vi "String2Array.vi"(7 "dimension size":i32=6, 10 "String":string) -> (2 "Array":dbl[](array[numeric]))   [LabVIEW 2013]
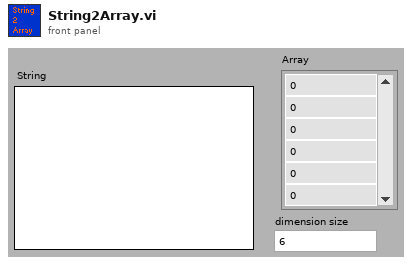
[diagram p1: front panel]
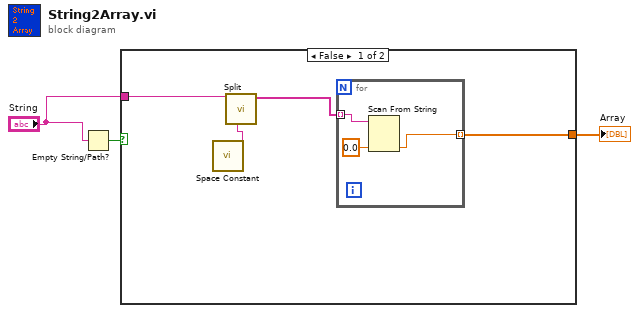
[diagram p0: block diagram]
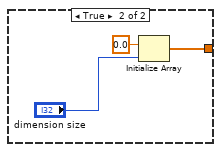
[diagram p2: hidden frame]
diagram:
  n1 = Empty String/Path?(string/path="String") -> (empty?=w3:bool)
  n2 = case shown="False" w3 {
    tunnel: "String" -> [w7 _]
    tunnel: [w4 w13] -> w1
    frame False {
      n3 = call <vilib>:"Space Constant.vi"() -> ("String"=w6:string)
      n4 = call "Split.vi"("delimiter"=w6, "String"=w7) -> ("Array Result"=w5:string[])  [unwired: 9 in]
      n5 = for {
        tunnel: w5 -> [w10] mode=indexing
        tunnel: [w9] -> w4 mode=indexing
        n6 = Scan From String(input string=w10, default 1=0.0 ("default value 1")) -> (output 1=w9:dbl)  [unwired: 3 in, 3 out]
      }
    }
    frame True {
      n7 = Initialize Array(0.0 ("element"), "dimension size") -> (w13:dbl[])
    }
  }
  "Array" <- w1
